vi "multi_set_Benchmark.vi"() -> ()   [LabVIEW 2017]
uses:
  SoftmotionClass/SoftmotionAxis/SoftmotionAxis.lvclass
  Utilities/StateMachine.ctl
  Utilities/Clear.vi
  Utilities/Set.vi
  <vilib>/NI_Real-Time Target Support.lvlib
  Utilities/Bit Manipulation.lvlib
  Utilities/WordManipulationLibrary.lvlib
panel:
  in  "Data_in":u16 format="%08b"
  out "Array":T1[](array[typedef])
  out "appended array":dbl[](array[numeric])
  out "SoftmotionAxis out":refnum<class "SoftmotionAxis.lvclass">
  out "Mean time (us)":dbl format="%.3g"
  in  "Warmup iterations":i32=10
  in  "Calibrate?":bool
  out "Execution histogram":T2(graph)
  out "Standard deviation (us)":dbl format="%.3g"
  out "Max jitter (us)":dbl format="%.3g"
  out "Execution times (us)":dbl[](graph)
  in  "Iterations":i32=1000
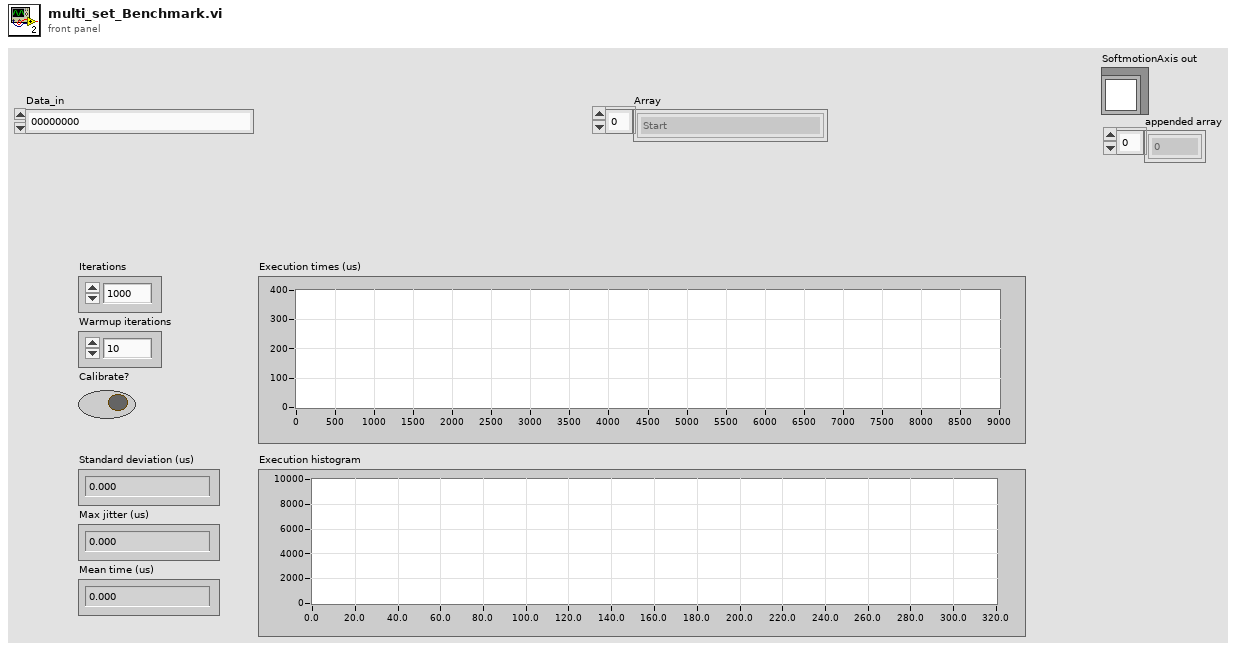
[diagram p1: front panel]
types:
  T1 = typedef "WordManipulationLibrary.lvlib/StateMachine.ctl" = enum16{"Start", "Not Ready to Switch On", "Switch On Disabled", "Ready to Switch On", "Switched On", "Operation enable", "Quick Stop Active", "Fault Reaction Active", "Fault"}
  T2 = cluster{"X Values":dbl[], "Histogram: h(x)":i32[]}
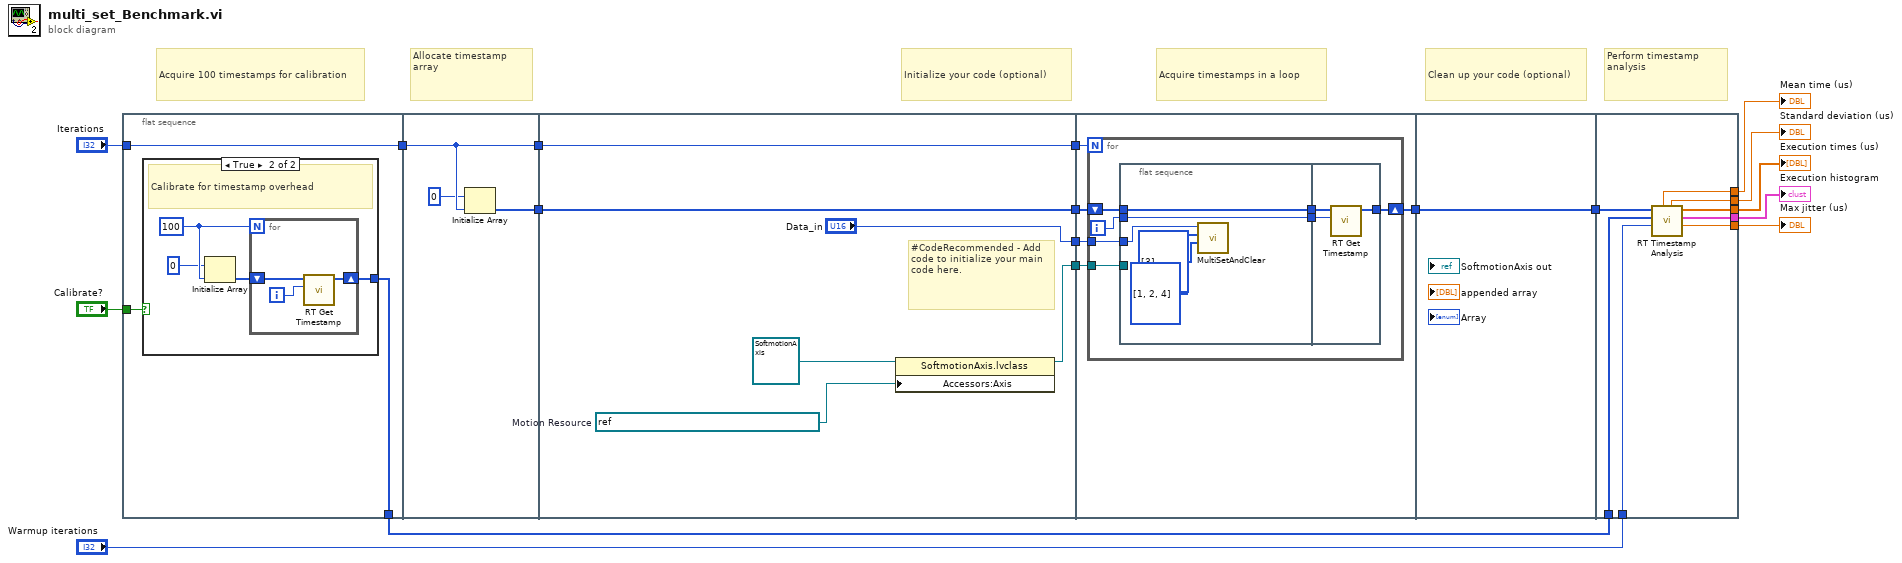
[diagram p0: block diagram]
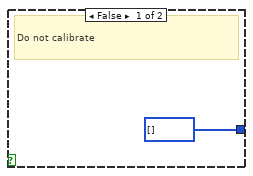
[diagram p2: hidden frame]
diagram:
  # "Perform timestamp analysis"
  # "Clean up your code (optional)"
  # "Acquire timestamps in a loop"
  # "Initialize your code (optional)"
  # "Allocate timestamp array"
  # "Acquire 100 timestamps for calibration"
  n1 = flat-sequence {
    tunnel: "Iterations" -> [w21]
    tunnel: [w21] -> w18
    tunnel: "Calibrate?" -> [w20]
    tunnel: [w19] -> w9
    tunnel: [w31] -> w17
    tunnel: [w32] -> w16
    tunnel: w18 -> [w31]
    tunnel: [w38] -> w15
    tunnel: [w37] -> w14
    tunnel: w17 -> [w38]
    tunnel: w16 -> [w37]
    tunnel: [w34] -> w2
    tunnel: ["Data_in"] -> w1
    tunnel: [w43] -> w13
    tunnel: w15 -> [w42]
    tunnel: w14 -> [w41]
    tunnel: w2 -> [w40]
    tunnel: w1 -> [w39]
    tunnel: w13 -> [w59]
    tunnel: [w59] -> w12
    tunnel: w12 -> [w67]
    tunnel: w9 -> [w66]
    tunnel: [w65] -> w3
    tunnel: [w64] -> w7
    tunnel: [w63] -> w6
    tunnel: [w62] -> w8
    tunnel: "Warmup iterations" -> [w61]
    tunnel: [w60] -> w4
    frame #0 {
      n2 = case shown="True" w20 {
        tunnel: [u64[] [] w26] -> w19
        frame False {
          # "Do not calibrate"
        }
        frame True {
          w24 = 100
          # "Calibrate for timestamp overhead"
          n3 = Initialize Array(u64 0, w24) -> (w25:u64[])
          n4 = for {
            N: w24 -> [_]
            shift-right: [w27] -> w26
            shift-left: w25 -> [w28]
            i -> [w29]
            n5 = call <vilib>:"RT Get Timestamp.vi"("iteration"=w29, "timestamp array in"=w28) -> ("timestamp array out"=w27:u64[])  [unwired: 1 in, 8 out]
          }
        }
      }
    }
    frame #1 {
      n6 = Initialize Array(u64 0, w31) -> (w32:u64[])
    }
    frame #2 {
      w35 = refnum<k21> "nism://RT CompactRIO Target/Axis 1"  # Motion Resource
      # "#CodeRecommended - Add code to initialize your main code here."
      n7 = property class="SoftmotionAxis.lvclass"(reference=refnum<class "SoftmotionAxis.lvclass"> refnum ("SoftmotionAxis.lvclass"), "Accessors:Axis"=w35) -> (reference out=w34:refnum<class "SoftmotionAxis.lvclass">)  [unwired: 1 in, 1 out]
    }
    frame #3 {
      n8 = for {
        N: w42 -> [_]
        shift-right: [w50] -> w43
        shift-left: w41 -> [w49]
        tunnel: w40 -> [w45]
        tunnel: w39 -> [w44]
        i -> [w48]
        n9 = flat-sequence {
          tunnel: w49 -> [w55]
          tunnel: [w55] -> w47
          tunnel: w48 -> [w54]
          tunnel: [w54] -> w46
          tunnel: w45 -> [_]
          tunnel: w44 -> [w53]
          tunnel: [w58] -> w50
          tunnel: w47 -> [w56]
          tunnel: w46 -> [w57]
          frame #0 {
            n10 = call "MultiSetAndClear.vi"("Bits_To_Clear"=u8[] [3], "Bits_To_Set"=u8[] [1, 2, 4], "Data_in"=w53) -> ()  [unwired: 8 in, 1 out]
          }
          frame #1 {
            n11 = call <vilib>:"RT Get Timestamp.vi"("iteration"=w57, "timestamp array in"=w56) -> ("timestamp array out"=w58:u64[])  [unwired: 1 in, 8 out]
          }
        }
      }
    }
    frame #4 {
    }
    frame #5 {
      n12 = call <vilib>:"RT Timestamp Analysis.vi"("warmup iterations"=w61, "calibration array"=w66, "timestamp array"=w67) -> ("max jitter (uS)"=w64:dbl, "execution histogram"=w65:T2, "execution times (uS)"=w62:dbl[], "standard deviation (uS)"=w63:dbl, "mean time (uS)"=w60:dbl)  [unwired: 1 in, 3 out]
    }
  }
  "Execution times (us)" <- w8
  "Max jitter (us)" <- w7
  "Standard deviation (us)" <- w6
  "Execution histogram" <- w3
  "Mean time (us)" <- w4
